vi "Acquire loop.vi"(8 "error in (no error)":errorcluster, 10 "notifier in":refnum<notifier>, 11 "Queue in":refnum<queue>) -> ()   [LabVIEW 2015]
uses:
  TypeDefs/Queue Data.ctl
  App Data.vi
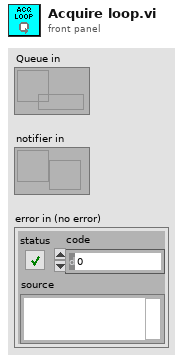
[diagram p1: front panel]
types:
  T1 = typedef "Queue Data.ctl" = cluster{"Action":string}
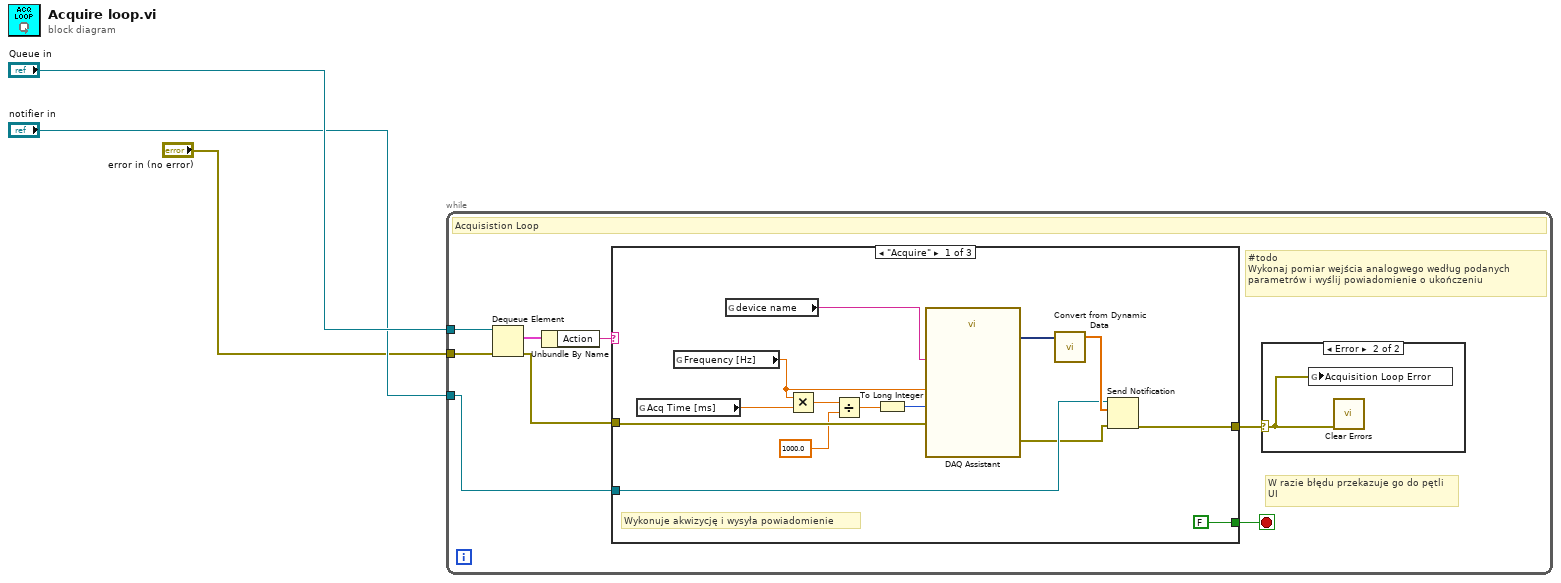
[diagram p0: block diagram]
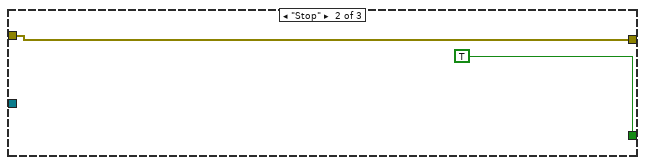
[diagram p3: hidden frame]
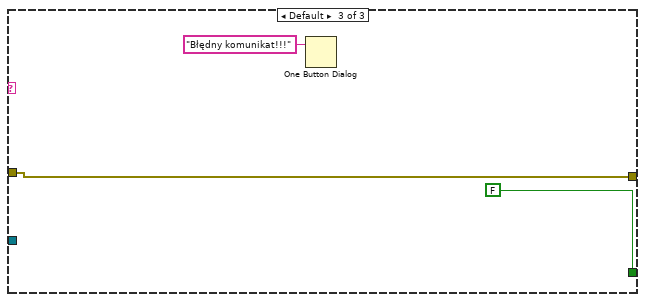
[diagram p4: hidden frame]
diagram:
  n1 = while {
    tunnel: "error in (no error)" -> [w9]
    tunnel: "Queue in" -> [w8]
    tunnel: "notifier in" -> [w4]
    stop <- w6 stop-if-true
    # "#todo\nWykonaj pomiar wejścia analogwego według podanych \nparametrów i wyślij powiadomienie o ukończeniu"
    # "W razie błędu przekazuje go do pętli\nUI"
    # "Acquisistion Loop"
    n2 = Dequeue Element(queue=w8, error in (no error)=w9) -> (element=w11:T1, error out=w7:errorcluster)  [unwired: 1 in, 2 out]
    n3 = Unbundle By Name(w11) -> ("Action"=w10:string)
    n4 = case shown="\"Acquire\"" w10 {
      tunnel: w7 -> [w21 w27 w30]
      tunnel: [FALSE TRUE FALSE] -> w6
      tunnel: [w14 w27 w30] -> w5
      tunnel: w4 -> [w15 _ _]
      frame "Acquire" {
        # "Wykonuje akwizycję i wysyła powiadomienie"
        n5 = global read "App Data.vi" "Acq Time [ms]"() -> (w24:dbl)
        n6 = global read "App Data.vi" "Frequency [Hz]"() -> (w23:dbl)
        n7 = global read "App Data.vi" "device name"() -> (w25:tag)
        n8 = Multiply(x=w23, y=w24) -> (x*y=w22:dbl)
        n9 = Divide(x=w22, y=1000.0) -> (x/y=w19:dbl)
        n10 = To Long Integer(number=w19) -> (32bit integer=w18:i32)
        n11 = call "DAQ Assistant"("rate"=w23, "number of samples"=w18, "error in"=w21, "device name"=w25) -> ("data"=w17:dynamicdata, "error out"=w13:errorcluster)  [unwired: 13 in, 1 out]
        n12 = call "Convert from Dynamic Data"("Dynamic Data Type"=w17) -> ("Array"=w16:dbl[])  [unwired: 3 in]
        n13 = Send Notification(notification=w16, notifier=w15, error in (no error)=w13) -> (error out=w14:errorcluster)  [unwired: 1 out]
      }
      frame "Stop" {
      }
      frame Default {
        n14 = One Button Dialog(message="Błędny komunikat!!!") -> ()  [unwired: 1 in, 1 out]
      }
    }
    n15 = case shown="Error" w5 {
      selector: w5 -> [_ w12]
      frame No Error {
      }
      frame Error {
        n16 = global write "App Data.vi" "Acquisition Loop Error"(w12) -> ()
        n17 = call <vilib>:"Clear Errors.vi"("error in (no error)"=w12) -> ()  [unwired: 5 in, 2 out]
      }
    }
  }
